vi "GetText.vi"(8 "error in":errorcluster, 11 "Abstract Channel in":refnum<class "Abstract Channel.lvclass">) -> (0 "error out":errorcluster, 1 "additional text":string, 2 "text":string, 3 "Abstract Channel out":refnum<class "Abstract Channel.lvclass">, 4 "glyph":string)   [LabVIEW 2025, in "Abstract Engine.lvlib" / "Abstract Channel.lvclass"]
doc: "Returns the text representation of the node used for the tree control.Copyright 2017 National Instruments Corporation\n\nLicensed under the Apache License, Version 2.0 (the \"License\"); you may not use this file except in compliance with the License. You may obtain a copy of the License at http://www.apache.org/licenses/LICENSE-2.0\nUnless required by applicable law or agreed to in writing, software distributed under the License is distributed on an \"AS IS\" BASIS, WITHOUT WARRANTIES OR CONDITIONS OF ANY KIND, either express or implied. See the License for the specific language governing permissions and limitations under the License."
uses:
  Abstract Channel.lvclass
  Abstract Channel.lvclass/Abstract Channel.ctl
  Channel configuration/Channel configuration.lvclass/Channel configuration.ctl
  Channel configuration/Read Channel Setting.vi
  Channel configuration/Channel configuration.lvclass
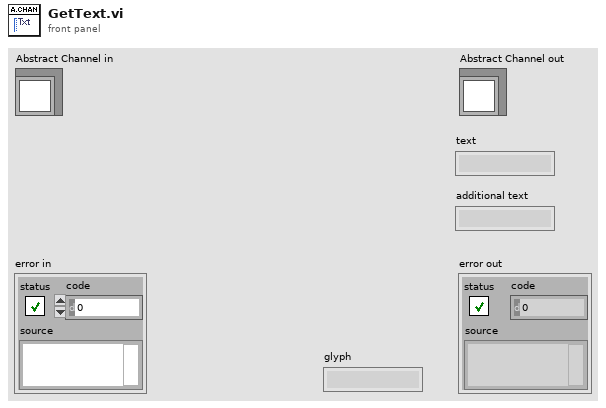
[diagram p1: front panel]
types:
  T1 = typedef "Abstract Engine.lvlib/Channel configuration.lvclass/Default Channel.ctl" = cluster{"Address":string, "SW Alias":string, "Description":string, "Enabled":bool, "Node Class":string}
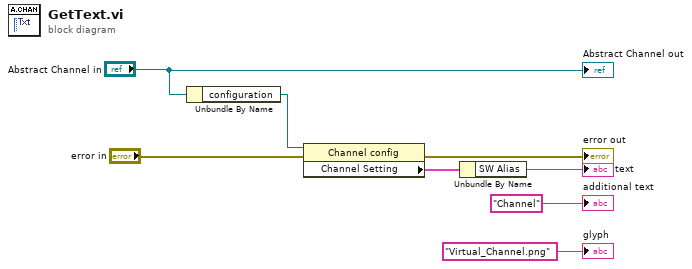
[diagram p0: block diagram]
diagram:
  n1 = Unbundle By Name("Abstract Channel in") -> ("configuration"=w3:refnum<class "Channel configuration.lvclass">)
  n2 = property class="Channel config"(reference=w3, error in="error in") -> (error out=→"error out":errorcluster, "Channel Setting"=w2:T1)  [unwired: 1 out]
  n3 = Unbundle By Name(w2) -> ("SW Alias"=→"text":string)
  "Abstract Channel out" <- "Abstract Channel in"
  "additional text" <- "Channel" ("additional text")
  "glyph" <- "Virtual_Channel.png" ("glyph")
